vi "ICM Open Initializer.vi"(8 "error in (no error)":errorcluster, 11 "ICM File In":path) -> (0 "error out":errorcluster, 3 "Init out":refnum<class "Initialize.lvclass">)   [LabVIEW 2018]
doc: "ICM Open Bus.vi\n\nThis VI finds the Bus of the current configuration file, opens the object, and reads its configuration data.\n\nInstrument Communication Module Version 1.0\nSeptember, 2017 Original Code Consulting David Thomson\n www.originalcode.com"
uses:
  Initialize/Initialize.lvclass
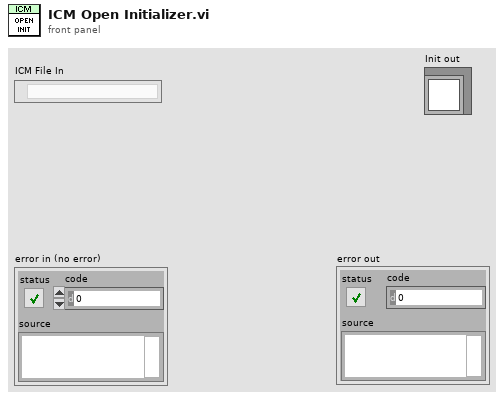
[diagram p1: front panel]
types:
  T1 = enum32{"invalid app kind", "Development System", "Run Time System", "Student Edition", "Embedded LabVIEW", "Evaluation", "Custom"}
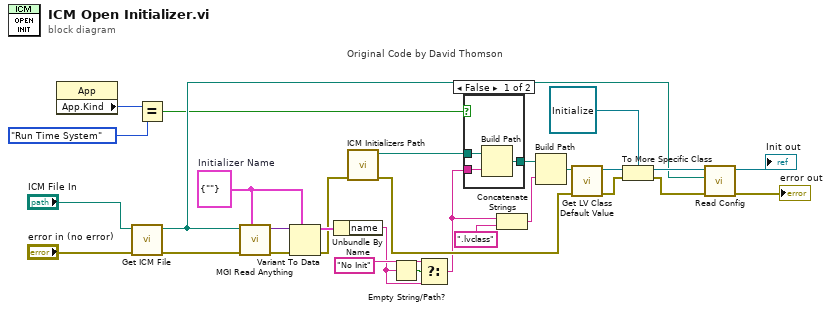
[diagram p0: block diagram]
diagram:
  w27 = cluster{"name":string} {"name"=""}  # Initializer Name
  n1 = property class="App"() -> ("App.Kind"=w10:T1)  [unwired: 2 in, 2 out]
  n2 = call "Get ICM File.vi"("error in (no error)"="error in (no error)", "ICM File In"="ICM File In") -> ("error out"=w20:errorcluster, "ICM File"=w15:path)  [unwired: 8 in]
  n3 = Equal?(x=w10, y=T1."Run Time System" ("Application:Kind")) -> (x = y?=w8:bool)
  n4 = call <userlib>:"MGI Read Anything.vi"("Type of Anything"=w27, "Error In"=w20, "Path (dialog)"=w15) -> ("Error Out"=w29:errorcluster, "Anything"=w28:variant)  [unwired: 5 in, 2 out]
  n5 = Variant To Data(error in=w29, type=w27, Variant=w28) -> (data=w23:cluster{"name":string}, error out=w13:errorcluster)
  n6 = Unbundle By Name(w23) -> ("name"=w2:string)
  n7 = call "ICM Initializers Path.vi"("error in (no error)"=w13) -> ("error out"=w14:errorcluster, "ICM Queries Path"=w11:path)  [unwired: 9 in]
  n8 = Empty String/Path?(string/path=w2) -> (empty?=w4:bool)
  n9 = Select(t="No Init", s=w4, f=w2) -> (s? t:f=w1:string)
  n10 = case "Original Code by David Thomson" shown="False" w8 {
    tunnel: w11 -> [w32 w33]
    tunnel: [w31 w33] -> w12
    tunnel: w1 -> [w30 _]
    frame False {
      n11 = Build Path(base path=w32, name or relative path=w30) -> (appended path=w31:path)
    }
    frame True {
    }
  }
  n12 = Concatenate Strings(w1, ".lvclass" ("string")) -> (w24:string)
  n13 = Build Path(base path=w12, name or relative path=w24) -> (appended path=w26:path)
  n14 = call <vilib>:"Get LV Class Default Value.vi"("error in (no error)"=w14, "class path"=w26) -> ("error out"=w22:errorcluster, "object"=w21:refnum<class>)  [unwired: 8 in]
  n15 = To More Specific Class(target class=refnum<class "Initialize.lvclass"> refnum ("Init out 2"), reference=w21, error in=w22) -> (specific class reference=w18:refnum<class "Initialize.lvclass">, error out=w17:errorcluster)
  n16 = call-dynamic "Read Config.vi"("error in (no error)"=w17, "ICM File In"=w15, "Init in"=w18) -> ("error out"=→"error out":errorcluster, "Init out"=→"Init out":refnum<class "Initialize.lvclass">)  [unwired: 7 in]
